vi "Read GIF File (Animated).vi"(8 "error in (no error)":errorcluster, 11 "path to GIF file":path) -> (0 "error out":errorcluster, 1 "animated?":bool, 2 "images data":T1[](array[typedef]), 3 "path":path, 4 "Delay (ms)":u32[](array[numeric]))   [LabVIEW 2020, in "openg_picture.lvlib" / "gif.lvlib"]
doc: "Reads a multi-frame (animated) Compuserve GIF file. If no path is specified, a file dialog is used to find the file."
uses:
  <vilib>/picture/picture.llb/imagedata.ctl
  gif.lvlib
panel:
  # "Read GIF File (Animated).vi\n\nReads a multi-frame (animated) Compuserve GIF file. If no path is specified, a file dialog is used to find the file.\n\nPlease visit http://www.OpenG.org to learn about the\nOpen Source LabVIEW software movement.\n\nNOTICE -- YOU MUST LEAVE THIS NOTICE IN PLACE.  PER THE TERMS OF THE LICENSE BELOW, YOU MAY SUBLICENSE THIS SOFTWARE \nIN ANY WAY THAT DOES NOT CONFLICT WITH THIS LICENSE.\n\n### BSD License (http://www.opensource.org/licenses/bsd-license.php) Begin ###\n \nCopyright (c) 2007, Bill Clench <bclench@yahoo.com>\n\nAll rights reserved.\n\nRedistribution and use in source and binary forms, with or without modification, are permitted provided that the following conditions are met:\n\n    * Redistributions of source code must retain the above copyright notice, this list of conditions and the following disclaimer.\n    * Redistributions in binary form must reproduce the above copyright notice, this list of conditions and the following disclaimer in the \n       documentation and/or other materials provided with the distribution.\n    * Neither the name of SciWare, James Kring, Inc., nor the names of its contributors may be used to endorse or promote products derived \n       from this software without specific prior written permission.\n\nTHIS SOFTWARE IS PROVIDED BY THE COPYRIGHT HOLDERS AND CONTRIBUTORS \"AS IS\" AND ANY EXPRESS OR IMPLIED WARRANTIES, \nINCLUDING, BUT NOT LIMITED TO, THE IMPLIED WARRANTIES OF MERCHANTABILITY AND FITNESS FOR A PARTICULAR PURPOSE ARE \nDISCLAIMED. IN NO EVENT SHALL THE COPYRIGHT OWNER OR CONTRIBUTORS BE LIABLE FOR ANY DIRECT, INDIRECT, INCIDENTAL,\n SPECIAL, EXEMPLARY, OR CONSEQUENTIAL DAMAGES (INCLUDING, BUT NOT LIMITED TO, PROCUREMENT OF SUBSTITUTE GOODS OR \nSERVICES; LOSS OF USE, DATA, OR PROFITS; OR BUSINESS INTERRUPTION) HOWEVER CAUSED AND ON ANY THEORY OF LIABILITY, \nWHETHER IN CONTRACT, STRICT LIABILITY, OR TORT (INCLUDING NEGLIGENCE OR OTHERWISE) ARISING IN ANY WAY OUT OF THE USE \nOF THIS SOFTWARE, EVEN IF ADVISED OF THE POSSIBILITY OF SUCH DAMAGE.\n\n### BSD License End ###"
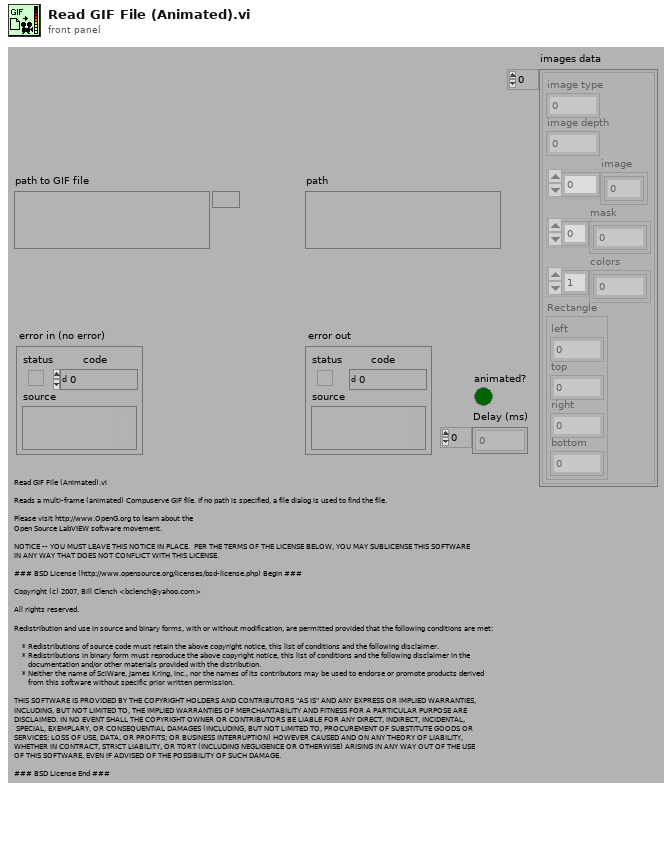
[diagram p1: front panel]
types:
  T1 = typedef "imagedata.ctl" = cluster{"image type":i32, "image depth":i32, "image":u8[], "mask":u8[], "colors":u32[], "Rectangle":cluster{"left":i16, "top":i16, "right":i16, "bottom":i16}}
  T2 = enum32{"existing file", "new file", "new or existing file", "existing dir", "new dir", "new or existing dir", "existing file (use LLBs)", "new file (use LLBs)", "new or existing file (use LLBs)", "new or existing file or directory (use LLBs)", "existing dir (use LLBs)", "new dir (use LLBs)", "new or existing dir (use LLBs)", "existing file or dir", "new file or dir", "new or existing file or dir", "existing file or dir (use LLBs)", "new file or dir (use LLBs)"}
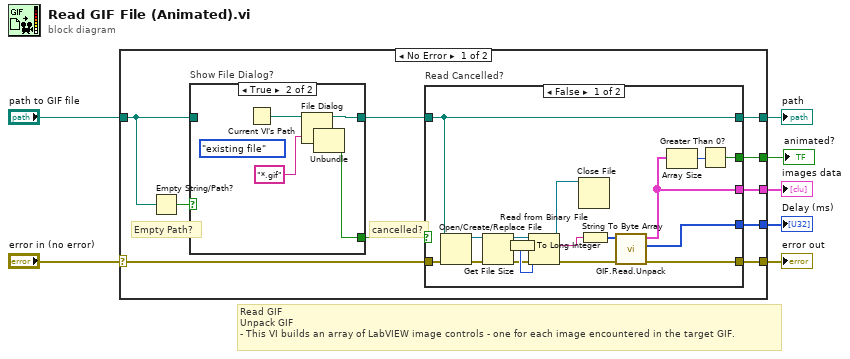
[diagram p0: block diagram]
diagram:
  # "Read GIF\nUnpack GIF\n- This VI builds an array of LabVIEW image controls - one for each image encountered in the target GIF."
  n1 = case shown="No Error" "error in (no error)" {
    selector: "error in (no error)" -> [w12 w44]
    tunnel: [w17 w44] -> w7
    tunnel: [w16 _] -> w6
    tunnel: "path to GIF file" -> [w13 w43]
    tunnel: [w11 w43] -> w3
    tunnel: [w10 _] -> w2
    tunnel: [w9 _] -> w1
    frame No Error {
      # "Empty Path?"
      # "cancelled?"
      n2 = Empty String/Path?(string/path=w13) -> (empty?=w15:bool)
      n3 = case "Show File Dialog?" shown="True" w15 {
        tunnel: [_ w23] -> w8
        tunnel: [w18 w20] -> w14
        tunnel: w13 -> [w18 _]
        frame False {
        }
        frame True {
          (unwired) T2."existing file" ("select mode (2)")
          n4 = Current VI's Path() -> (path=w21:path)
          n5 = File Dialog(6:"*.gif", 11:w21) -> (0:w19:errorcluster, 1:w23:bool, 3:w20:path)  [unwired: 5 in, 1 out]
          n6 = Unbundle(w19) -> ()  [unwired: 3 out]
        }
      }
      n7 = case "Read Cancelled?" shown="False" w8 {
        tunnel: w12 -> [w33 w42]
        tunnel: [w39 w42] -> w17
        tunnel: [w37 _] -> w16
        tunnel: w14 -> [w34 w41]
        tunnel: [w34 w41] -> w11
        tunnel: [w38 _] -> w10
        tunnel: [w35 _] -> w9
        frame False {
          n8 = Open/Create/Replace File(file path (use dialog)=w34, error in=w33) -> (refnum out=w28:refnum<file>, error out=w29:errorcluster)  [unwired: 4 in, 1 out]
          n9 = Get File Size(file=w28, error in=w29) -> (refnum out=w25:refnum<file>, size (in bytes)=w24:i64, 0:w26:errorcluster)
          n10 = To Long Integer(number=w24) -> (32bit integer=w27:i32)
          n11 = Read from Binary File(8:w26, 10:w27, 11:w25) -> (0:w30:errorcluster, 2:w32:string, 3:w31:refnum<file>)  [unwired: 3 in, 1 out]
          n12 = Close File(refnum=w31) -> ()  [unwired: 1 in, 2 out]
          n13 = String To Byte Array(string=w32) -> (unsigned byte array=w40:u8[])
          n14 = call "GIF.Read.Unpack.vi"("error in (no error)"=w30, "Raw GIF89a bytes"=w40) -> ("error out"=w39:errorcluster, "Delay (ms)"=w38:u32[], "Picture Array"=w37:T1[])  [unwired: 5 in]
          n15 = Array Size(array=w37) -> (size(s)=w36:i32)
          n16 = Greater Than 0?(x=w36) -> (x > 0?=w35:bool)
        }
        frame True {
        }
      }
    }
    frame Error {
    }
  }
  "error out" <- w7
  "images data" <- w6
  "path" <- w3
  "Delay (ms)" <- w2
  "animated?" <- w1
